vi "Load config.vi"(3 "error in (no error)":errorcluster) -> (7 "DAQ config params":T2={"DAQ Device Name"="Dev2", "Physical channel"=""}, 8 "FCR config params":T1={"VISA resource"="", "baud rate"=9600}, 10 "error out":errorcluster)   [LabVIEW 2020]
uses:
  controls/DAQ config parameters -- cluster.ctl
  controls/FCR config parameters -- cluster.ctl
  <vilib>/Utility/config.llb/Read Key (String).vi
  <vilib>/Utility/config.llb/NI_LVConfig.lvlib
  <vilib>/Utility/config.llb/Read Key (U32).vi
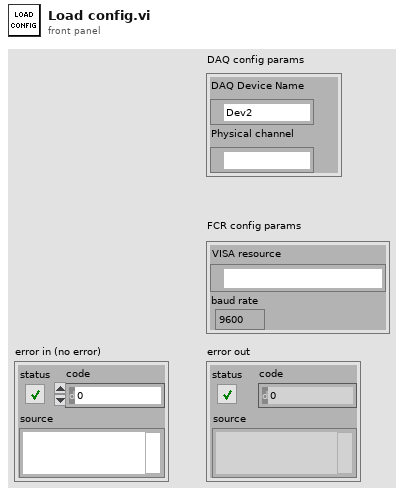
[diagram p1: front panel]
types:
  T1 = typedef "FCR config parameters -- cluster.ctl" = cluster{"VISA resource":refnum<visa-resource-name>, "baud rate":u32}
  T2 = typedef "DAQ config parameters -- cluster.ctl" = cluster{"DAQ Device Name":tag, "Physical channel":tag}
  T3 = typedef "NI_LVConfig.lvlib/Config Data RefNum.ctl" = refnum<k1>
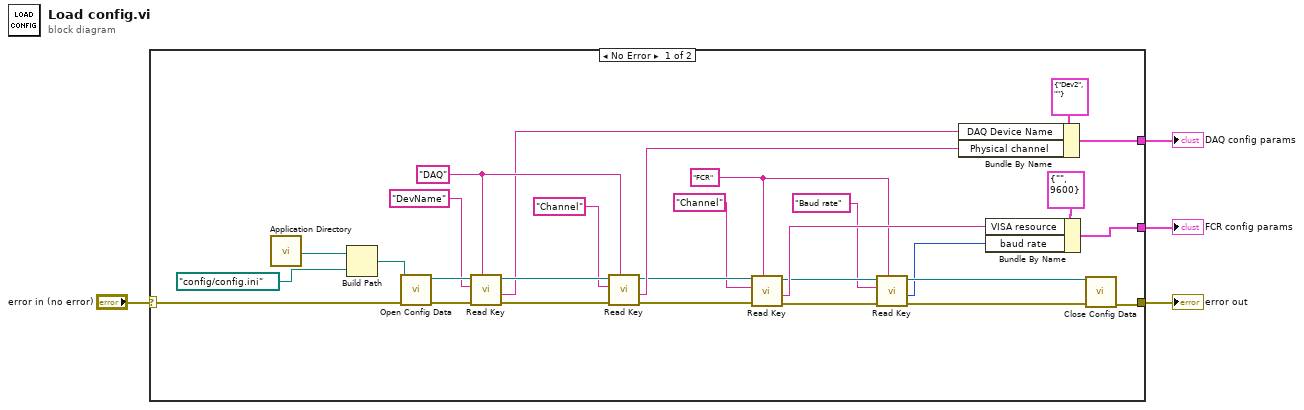
[diagram p0: block diagram]
diagram:
  n1 = case shown="No Error" "error in (no error)" {
    selector: "error in (no error)" -> [w30 w34]
    tunnel: [w23 w34] -> w3
    tunnel: [w18 _] -> w2
    tunnel: [w12 _] -> w1
    frame No Error {
      w6 = "FCR" ("section")
      w24 = "DAQ" ("section")
      n2 = call <vilib>:"Application Directory.vi"() -> ("Application Directory"=w33:path)
      n3 = Build Path(base path=w33, name or relative path=path "config/config.ini") -> (appended path=w31:path)
      n4 = call <vilib>:"Open Config Data.vi"("error in (no error)"=w30, "configuration file path"=w31) -> ("error out"=w29:errorcluster, "refnum"=w28:T3)  [unwired: 7 in, 1 out]
      n5 = call-poly <vilib>:"Read Key.vi"("section"=w24, "error in (no error)"=w29, "key"="DevName", "refnum"=w28) -> ("error out"=w26:errorcluster, "value"=w20:string, "refnum out"=w25:T3)  [unwired: 4 in, 1 out]
      n6 = call-poly <vilib>:"Read Key.vi"("section"=w24, "error in (no error)"=w26, "key"="Channel", "refnum"=w25) -> ("error out"=w16:errorcluster, "value"=w19:string, "refnum out"=w17:T3)  [unwired: 4 in, 1 out]
      n7 = call-poly <vilib>:"Read Key.vi"("section"=w6, "error in (no error)"=w16, "key"="Channel", "refnum"=w17) -> ("error out"=w11:errorcluster, "value"=w13:string, "refnum out"=w10:T3)  [unwired: 4 in, 1 out]
      n8 = call-poly <vilib>:"Read Key.vi"("section"=w6, "error in (no error)"=w11, "key"="Baud rate", "refnum"=w10) -> ("error out"=w8:errorcluster, "value"=w5:u32, "refnum out"=w9:T3)  [unwired: 4 in, 1 out]
      n9 = Bundle By Name(cluster=T2 {"DAQ Device Name"="Dev2", "Physical channel"=""} ("DAQ config params"), "DAQ Device Name"=w20, "Physical channel"=w19) -> (w18:T2)
      n10 = Bundle By Name(cluster=T1 {"VISA resource"="", "baud rate"=9600} ("FCR config params"), "VISA resource"=w13, "baud rate"=w5) -> (w12:T1)
      n11 = call <vilib>:"Close Config Data.vi"("error in (no error)"=w8, "refnum"=w9) -> ("error out"=w23:errorcluster)  [unwired: 8 in, 1 out]
    }
    frame Error {
    }
  }
  "error out" <- w3
  "DAQ config params" <- w2
  "FCR config params" <- w1
